vi "Query Frequency.vi"(8 "error in (no error)":errorcluster, 10 "Channel (0: Channel 1)":T1 items=["Channel 1", "Channel 2"], 11 "VISA resource name":refnum<visa-resource-name>) -> (0 "error out":errorcluster, 1 "frequency":dbl[unit], 3 "VISA resource name out":refnum<visa-resource-name>)   [LabVIEW 2015, in "Tektronix AFG 3000 Series.lvlib"]
doc: "Queries the frequency of a Tektronix AFG 3000 series function generator. May not be used when the run mode is set to sweep."
uses:
  Tektronix AFG 3000 Series.lvlib
  controls.llb/Channel.ctl
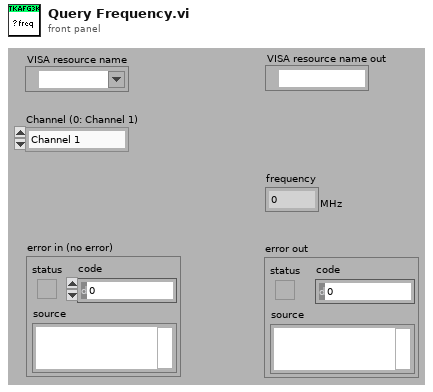
[diagram p1: front panel]
types:
  T1 = typedef "Channel.ctl" = u16
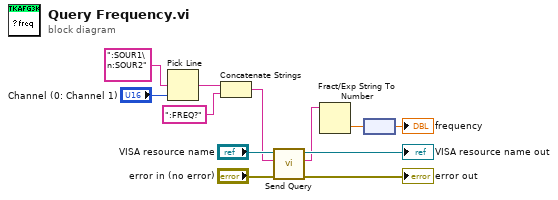
[diagram p0: block diagram]
diagram:
  n1 = Pick Line(multi-line string=":SOUR1\n:SOUR2", line index="Channel (0: Channel 1)") -> (output string=w9:string)  [unwired: 1 out]
  n2 = Concatenate Strings(w9, ":FREQ?" ("format string")) -> (w8:string)
  n3 = call "Send Query.vi"("error in (no error)"="error in (no error)", "write buffer"=w8, "VISA resource name"="VISA resource name") -> ("error out"=→"error out":errorcluster, "read buffer"=w3:string, "VISA resource name out"=→"VISA resource name out":refnum<visa-resource-name>)  [unwired: 1 in, 5 out]
  n4 = Fract/Exp String To Number(string=w3) -> (number=w2:dbl)  [unwired: 4 out]
  n5 = node(w2) -> (→"frequency":dbl[unit])
